vi "grabber.vi"() -> ()   [LabVIEW 2010]
uses:
  status_enum.ctl
  type definitions/command_enum.ctl
  <vilib>/rvi/interface/nirviReadWriteControl/nirviReadWriteControl.xnode
  FPGA_VI_reference.ctl
  <vilib>/rvi/interface/common/niFpgaNodeNameForErrorReporting.ctl
  <vilib>/rvi/errors/niLvFpgaWhatHappensToTopLevelVI.ctl
  <vilib>/dex/Flush And Wait Empty Condition.ctl
  <vilib>/rvi/interface/nirviMethod/nirviMethod.xnode
  <vilib>/rvi/interface/nirviCloseFPGA/nirviCloseFPGA.xnode
  <vilib>/Utility/error.llb/Error Cluster From Error Code.vi
  <vilib>/rvi/errors/niLvFpgaAdjustHostInterfaceError.vi
  <vilib>/FPGAPlugInAG/Dynamic/niLvFpga_Close_Dynamic.vi
  NiFpgaLv.dll
panel:
  out "loop counter":i32
  in  "writer buffer size":i32=1000000 format="%.0e"
  in  "Close front-panel?":bool=TRUE
  out "pixel counter":i64
  out "data read":u64[](array[numeric])
  out "last command during acquisition":T1
  out "last command":T1
  out "state":T2
  out "FIFO overflow":bool
  out "error out":errorcluster
  # "Grabber.exe"
  # "Grabber.exe of FPGAWrapperDL120115Galvo\n\n\nAuthor: Dominik Langer\ncopyright: University of Zurich, Switzerland"
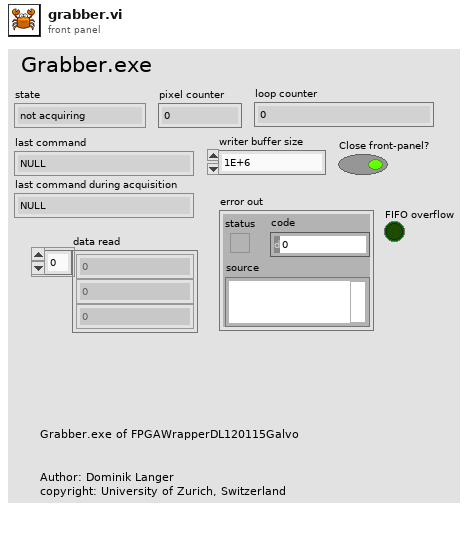
[diagram p1: front panel]
types:
  T1 = typedef "command_enum.ctl" = enum16{"NULL", "update", "start", "stop", "reset", "shut-down"}
  T2 = typedef "status_enum.ctl" = enum16{"not acquiring", "acquiring"}
  T3 = typedef "network_streaming_queues_cluster.ctl" = cluster{"configuration reader endpoint":refnum<k21>, "settings reader endpoint":refnum<k21>, "data writer endpoint":refnum<k21>, "command reader endpoint":refnum<k21>}
  T4 = typedef "FPGA_VI_reference.ctl" = refnum<k20>
  T5 = typedef "niFpgaNodeNameForErrorReporting.ctl" = enum16{"Open FPGA VI Reference", "Read/Write Control", "Invoke Method: Abort", "Invoke Method: Acknowledge IRQ", "Invoke Method: Download", "Invoke Method: FIFO.Configure", "Invoke Method: FIFO.Read", "Invoke Method: FIFO.Start", "Invoke Method: FIFO.Stop", "Invoke Method: FIFO.Write", "Invoke Method: Reset", "Invoke Method: Run", "Invoke Method: Wait on IRQ", "Close FPGA VI Reference"}
  T6 = typedef "niLvFpgaWhatHappensToTopLevelVI.ctl" = enum16{"top level VI scripted behind XNode", "top level VI inlined behind XNode"}
  T7 = typedef "settings_cluster.ctl" = cluster{"number of pixels":i32, "iterations per pixel":i32, "maximum bit-depth":i32, "pixel values cluster":T8, "triggered?":bool, "triggered flag valid?":bool, "gates":T9[]}
  T8 = typedef "channels_cluster.ctl" = cluster{"channel 0":u32, "channel 1":u32, "channel 2":u32, "channel 3":u32}
  T9 = typedef "gate_cluster.ctl" = cluster{"index":i32, "parameters":T10}
  T10 = typedef "gate_parameters_cluster.ctl" = cluster{"offset":i64, "pulsing":i64, "not pulsing":i64, "cycles per pulse":i64, "repetitions":i64}
  T11 = typedef "Flush And Wait Empty Condition.ctl" = u8
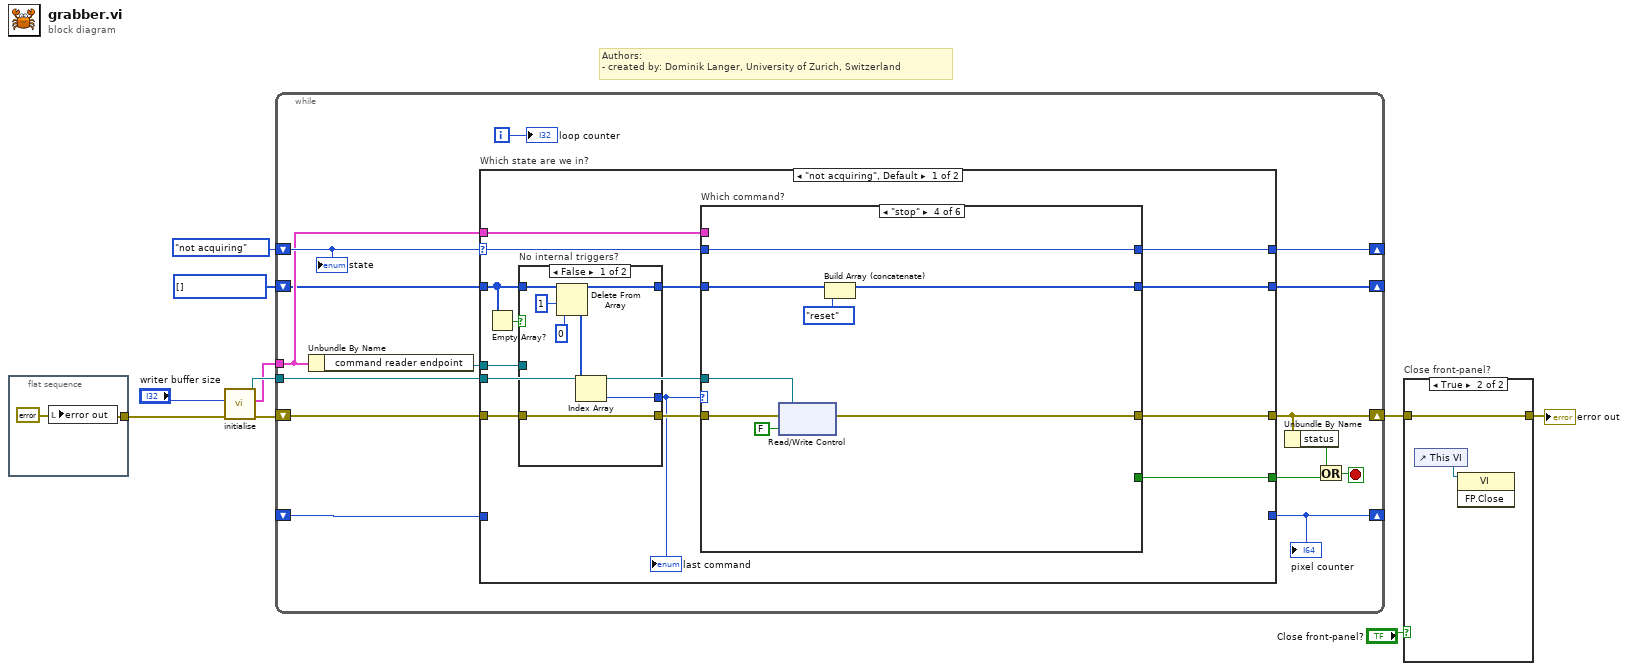
[diagram p0: block diagram]
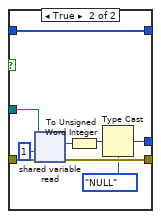
[diagram p2: hidden frame]
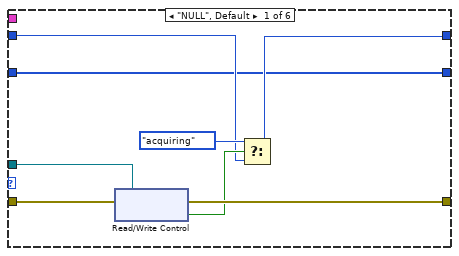
[diagram p3: hidden frame]
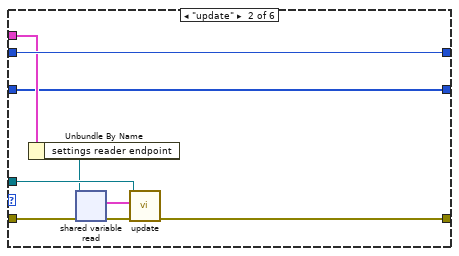
[diagram p4: hidden frame]
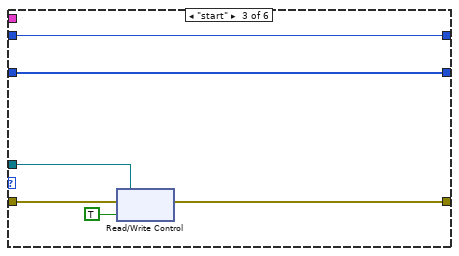
[diagram p5: hidden frame]
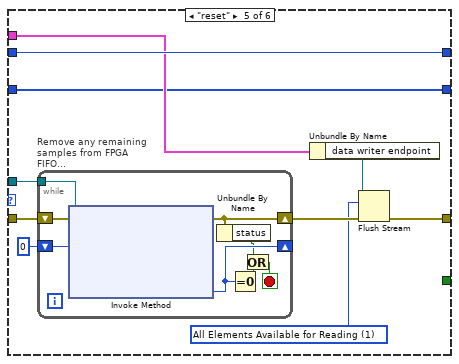
[diagram p6: hidden frame]
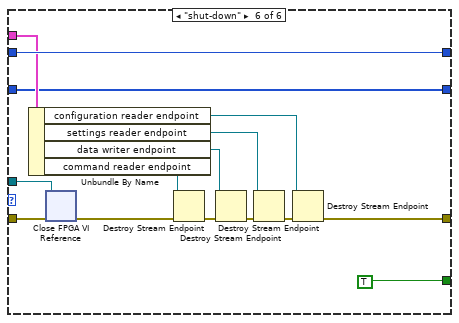
[diagram p7: hidden frame]
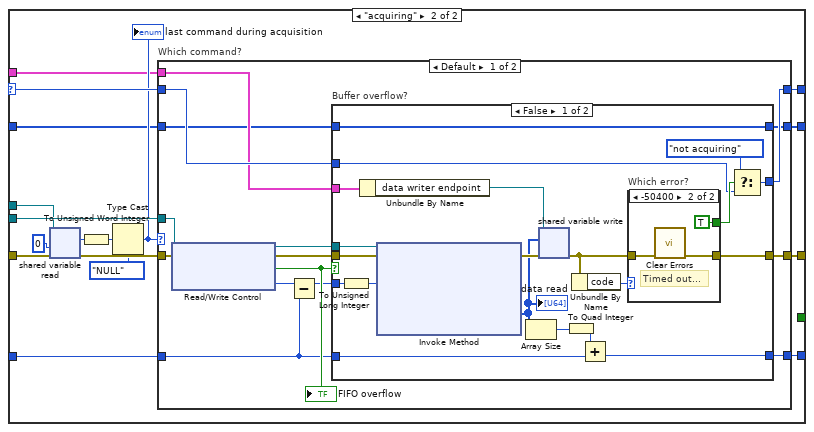
[diagram p8: hidden frame]
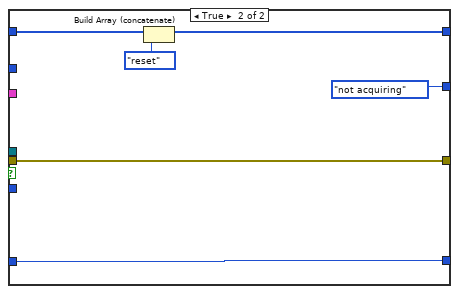
[diagram p10: hidden frame]
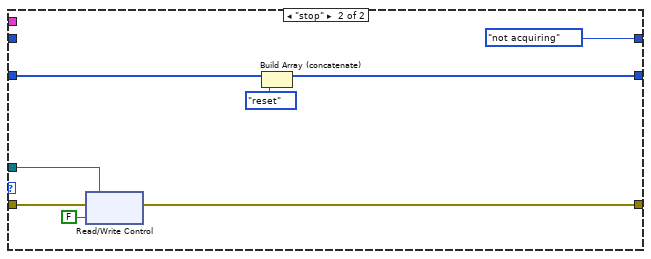
[diagram p11: hidden frame]
diagram:
  w1 = T1[] [] items=["NULL", "update", "start", "stop", "reset", "shut-down"]
  # "Authors: \n- created by: Dominik Langer, University of Zurich, Switzerland"
  n1 = flat-sequence {
    tunnel: [w11] -> w6
    frame #0 {
      w11 = errorcluster {"status"=FALSE, "code"=0, "source"=""} ("error in (no error)")
      n2 = local write "error out"(w11) -> ()
    }
  }
  n3 = call "initialise.vi"("error in (no error)"=w6, "writer buffer size"="writer buffer size") -> ("error out"=w5:errorcluster, "network streaming queues"=w2:T3, "FPGA VI Reference Out"=w3:T4)  [unwired: 7 in]
  n4 = while {
    shift-right: [w22] -> w7
    shift-left: w5 -> [w14]
    shift-right: [w24] -> _
    shift-left: status_enum."not acquiring" ("status") -> [w26]
    tunnel: w3 -> [w25]
    shift-right: [w18] -> _
    shift-left: _ -> [w23]
    tunnel: w2 -> [w16]
    shift-right: [w13] -> _
    shift-left: w1 -> [w12]
    i -> [w17]
    stop <- w19 stop-if-true
    n5 = Unbundle By Name(w16) -> ("command reader endpoint"=w15:refnum<k21>)
    n6 = case "Which state are we in?" shown="\"not acquiring\", Default" w26 {
      selector: w26 -> [w36 w335]
      tunnel: w14 -> [w39 w333]
      tunnel: [w40 w336] -> w22
      tunnel: w25 -> [w34 w337]
      tunnel: w15 -> [w31 w331]
      tunnel: [w35 w334] -> w24
      tunnel: w23 -> [_ w326]
      tunnel: [w33 _] -> w21
      tunnel: [_ w325] -> w18
      tunnel: w16 -> [w32 w324]
      tunnel: [w30 w322] -> w13
      tunnel: w12 -> [w28 w321]
      frame "not acquiring", Default {
        n7 = Empty Array?(array=w28) -> (empty?=w27:bool)
        n8 = case "No internal triggers?" shown="False" w27 {
          tunnel: w39 -> [w47 w54]
          tunnel: [w47 w53] -> w38
          tunnel: [w42 w52] -> w37
          tunnel: w31 -> [_ w51]
          tunnel: w28 -> [w46 w48]
          tunnel: [w41 w48] -> w29
          frame False {
            n9 = Delete From Array(array=w46, length=1, index=0) -> (deleted portion=w43:T1[], array with subset deleted=w41:T1[])
            n10 = Index Array(array=w43) -> (element=w42:T1)  [unwired: 1 in]
          }
          frame True {
            n11 = shared-variable-read(w51, w54, 1 ("timeout in ms (-1)")) -> (w53:errorcluster, w55:u32)  [unwired: 2 out]
            n12 = To Unsigned Word Integer(number=w55) -> (unsigned 16bit integer=w56:u16)
            n13 = Type Cast(type=command_enum."NULL" ("command"), x=w56) -> (*(type *) &x=w52:T1)
          }
        }
        "last command" <- w37
        n14 = case "Which command?" shown="\"stop\"" w37 {
          tunnel: w38 -> [w64 w115 w121 w167 w215 w311]
          tunnel: [w63 w112 w119 w166 w212 w308] -> w40
          tunnel: w36 -> [w60 w116 w118 w169 w218 w314]
          tunnel: [w59 w116 w118 w169 w218 w314] -> w35
          tunnel: w34 -> [w58 w111 w120 w165 w217 w312]
          tunnel: [_ _ _ _ _ TRUE] -> w33
          tunnel: w32 -> [_ w110 _ _ w211 w305]
          tunnel: w29 -> [w57 w108 w117 w164 w209 w300]
          tunnel: [w57 w108 w117 w162 w209 w300] -> w30
          frame "NULL", Default {
            n15 = xnode "Read/Write Control"("FPGA VI Reference In"=w58, "error in"=w64) -> ("error out"=w63:errorcluster, "acquiring?"=w62:bool)  [unwired: 1 out]
            n16 = Select(t=status_enum."acquiring" ("status"), s=w62, f=w60) -> (s? t:f=w59:T2)
          }
          frame "update" {
            n17 = Unbundle By Name(w110) -> ("settings reader endpoint"=w109:refnum<k21>)
            n18 = shared-variable-read(w109, w115) -> (w113:errorcluster, w114:T7)  [unwired: 1 in, 2 out]
            n19 = call "update.vi"("error in"=w113, "settings cluster"=w114, "FPGA VI ref"=w111) -> ("error out"=w112:errorcluster)  [unwired: 8 in]
          }
          frame "start" {
            n20 = xnode "Read/Write Control"("FPGA VI Reference In"=w120, "error in"=w121, "acquire"=TRUE) -> ("error out"=w119:errorcluster)  [unwired: 1 out]
          }
          frame "stop" {
            n21 = xnode "Read/Write Control"("FPGA VI Reference In"=w165, "error in"=w167, "acquire"=FALSE) -> ("error out"=w166:errorcluster)  [unwired: 1 out]
            n22 = Build Array (concatenate)(w164, command_enum."reset" ("command")) -> (w162:T1[])
          }
          frame "reset" {
            w210 = T11 1 items=["All Elements Read From Stream", "All Elements Available for Reading"] ("wait condition")
            n23 = while "Remove any remaining samples from FPGA FIFO..." {
              tunnel: w217 -> [w225]
              shift-right: [w223] -> _
              shift-left: u32 0 ("Elements Remaining") -> [w224]
              shift-right: [w222] -> w213
              shift-left: w215 -> [w226]
              stop <- w219 stop-if-true
              n24 = xnode "Invoke Method"("FPGA VI Reference In"=w225, "error in"=w226, "Number of Elements"=w224) -> ("error out"=w222:errorcluster, "Elements Remaining"=w223:u32)  [unwired: 1 in, 2 out]
              n25 = Unbundle By Name(w222) -> ("status"=w220:bool)
              n26 = Equal To 0?(x=w223) -> (x = 0?=w221:bool)
              n27 = Or(x=w220, y=w221) -> (x .or. y?=w219:bool)
            }
            n28 = Unbundle By Name(w211) -> ("data writer endpoint"=w214:refnum<k21>)
            n29 = Flush Stream(8:w213, 10:w210, 11:w214) -> (0:w212:errorcluster)  [unwired: 1 in, 2 out]
          }
          frame "shut-down" {
            n30 = Unbundle By Name(w305) -> ("configuration reader endpoint"=w301:refnum<k21>, "settings reader endpoint"=w302:refnum<k21>, "data writer endpoint"=w303:refnum<k21>, "command reader endpoint"=w304:refnum<k21>)
            n31 = xnode "Close FPGA VI Reference"("FPGA VI Reference In"=w312, "error in"=w311) -> ("error out"=w310:errorcluster)
            n32 = Destroy Stream Endpoint(8:w310, 11:w304) -> (0:w309:errorcluster)
            n33 = Destroy Stream Endpoint(8:w309, 11:w303) -> (0:w307:errorcluster)
            n34 = Destroy Stream Endpoint(8:w307, 11:w302) -> (0:w306:errorcluster)
            n35 = Destroy Stream Endpoint(8:w306, 11:w301) -> (0:w308:errorcluster)
          }
        }
      }
      frame "acquiring" {
        n36 = shared-variable-read(w331, w333, 0 ("timeout in ms (-1)")) -> (w332:errorcluster, w330:u32)  [unwired: 2 out]
        n37 = To Unsigned Word Integer(number=w330) -> (unsigned 16bit integer=w329:u16)
        n38 = Type Cast(type=command_enum."NULL" ("command"), x=w329) -> (*(type *) &x=w327:T1)
        "last command during acquisition" <- w327
        n39 = case "Which command?" shown="Default" w327 {
          tunnel: w337 -> [w350 w535]
          tunnel: [w349 w536] -> w336
          tunnel: w335 -> [w348 _]
          tunnel: [w347 status_enum."not acquiring" ("status")] -> w334
          tunnel: w332 -> [w346 w537]
          tunnel: w326 -> [w340 _]
          tunnel: [w344 _] -> w325
          tunnel: w324 -> [w341 _]
          tunnel: [w338 w532] -> w322
          tunnel: w321 -> [w339 w534]
          frame Default {
            n40 = xnode "Read/Write Control"("FPGA VI Reference In"=w350, "error in"=w346) -> ("FPGA VI Reference Out"=w351:T4, "error out"=w352:errorcluster, "FIFO overflow"=w345:bool, "current pixel no."=w343:i64)
            "FIFO overflow" <- w345
            n41 = Subtract(x=w343, y=w340) -> (x-y=w342:i64)
            n42 = case "Buffer overflow?" shown="False" w345 {
              tunnel: w352 -> [w372 w455]
              tunnel: w351 -> [w371 _]
              tunnel: [w369 w455] -> w349
              tunnel: w348 -> [w357 _]
              tunnel: [w355 status_enum."not acquiring" ("status")] -> w347
              tunnel: w340 -> [w365 w453]
              tunnel: [w364 w453] -> w344
              tunnel: w342 -> [w362 _]
              tunnel: w341 -> [w360 _]
              tunnel: w339 -> [w353 w452]
              tunnel: [w353 w450] -> w338
              frame False {
                n43 = To Unsigned Long Integer(number=w362) -> (unsigned 32bit integer=w361:u32)
                n44 = Unbundle By Name(w360) -> ("data writer endpoint"=w359:refnum<k21>)
                n45 = xnode "Invoke Method"("FPGA VI Reference In"=w371, "error in"=w372, "Number of Elements"=w361) -> ("error out"=w368:errorcluster, "Data"=w354:u64[])  [unwired: 1 in, 2 out]
                "data read" <- w354
                n46 = Array Size(array=w354) -> (size(s)=w366:i32)
                n47 = shared-variable-write(w359, w368, w354) -> (w367:errorcluster)  [unwired: 1 in, 2 out]
                n48 = To Quad Integer(1:w366) -> (0:w363:i64)
                n49 = Unbundle By Name(w367) -> ("code"=w370:i32)
                n50 = Add(x=w363, y=w365) -> (x+y=w364:i64)
                n51 = case "Which error?" shown="-50400" w370 {
                  tunnel: [w373 w375] -> w369
                  tunnel: w367 -> [w373 w376]
                  tunnel: [_ TRUE] -> w358
                  frame 0, Default {
                  }
                  frame -50400 {
                    # "Timed out..."
                    n52 = call <vilib>:"Clear Errors.vi"("error in (no error)"=w376) -> ("error out"=w375:errorcluster)  [unwired: 6 in]
                  }
                }
                n53 = Select(t=status_enum."not acquiring" ("status"), s=w358, f=w357) -> (s? t:f=w355:T2)
              }
              frame True {
                n54 = Build Array (concatenate)(w452, command_enum."reset" ("command")) -> (w450:T1[])
              }
            }
          }
          frame "stop" {
            n55 = xnode "Read/Write Control"("FPGA VI Reference In"=w535, "error in"=w537, "acquire"=FALSE) -> ("error out"=w536:errorcluster)  [unwired: 1 out]
            n56 = Build Array (concatenate)(w534, command_enum."reset" ("command")) -> (w532:T1[])
          }
        }
      }
    }
    "pixel counter" <- w18
    n57 = Unbundle By Name(w22) -> ("status"=w20:bool)
    n58 = Or(x=w20, y=w21) -> (x .or. y?=w19:bool)
    "state" <- w26
    "loop counter" <- w17
  }
  n59 = case "Close front-panel?" shown="True" "Close front-panel?" {
    tunnel: [w579 w580] -> w8
    tunnel: w7 -> [w579 w580]
    frame False {
    }
    frame True {
      n60 = control-ref of="This VI"() -> (w581:refnum<vi>)
      n61 = invoke class="VI" method="FP.Close"(reference=w581) -> ()  [unwired: 2 in, 3 out]
    }
  }
  "error out" <- w8
